vi "MGCC_StaEst_global.vi"() -> ()   [LabVIEW 2016]
panel:
  out "StaEst_An":dbl[][][](array[numeric])
  out "StaEst_Vn":dbl[][][](array[numeric])
  in  "Vbase":dbl
  in  "Slack_bus":dbl
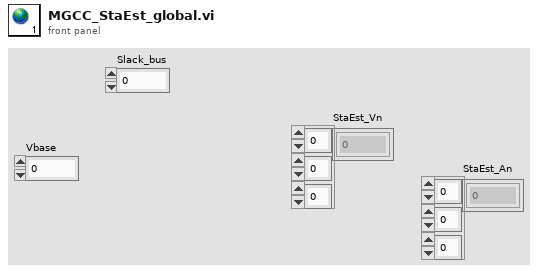
[diagram p1: front panel]
diagram:
